vi "Butterfly_PullDown RCV w_AWG.vi"(0 "Semiconductor Module Context":T2, 1 "RFPins":string[](array[string]), 2 "script name":string, 3 "R Thresholds":dbl[](array[numeric]), 4 "Capacitance":bool=TRUE, 5 "error in (no error)":errorcluster, 6 "VNAs Measurement Parameters":T1, 7 "Start_v":dbl=10.0 format="%#_13g", 8 "C_TH_Delta":dbl=2.0, 9 "Stop_v":dbl=41.0 format="%#_13g", 10 "Down_Butterfly_V_Sweep":dbl[](array[numeric]), 11 "Step_v":dbl=1.0, 12 "DOWNPublishNames":string[](array[string])) -> (14 "Semiconductor Module Context Out":T2, 19 "error out":errorcluster)   [LabVIEW 2013]
uses:
  <vilib>/NI_TestStand_SemiconductorModule/NI_TestStand_Semiconductor_Module.lvlibp/PinMap/General/SemiconductorModuleContext.ctl
  VNA/VNAs Measurement Parameters.ctl
  <instrlib>/niHSDIO/niHSDIO.llb/niHSDIO_ctl Trigger Script - trigID Values (Ring).ctl
  <instrlib>/niDCPower/nidcpower.llb/niDCPower Wait For Event - Event.ctl
  <vilib>/NI_TestStand_SemiconductorModule/NI_TestStand_Semiconductor_Module.lvlibp/PinMap/DC Power/PinsToNIDCPowerSessions.vi
  <vilib>/NI_TestStand_SemiconductorModule/NI_TestStand_Semiconductor_Module.lvlibp/PinMap/General/Publish/PublishDataDoubleFunctionalTest.vi
  <vilib>/NI_TestStand_SemiconductorModule/NI_TestStand_Semiconductor_Module.lvlibp/PinMap/General/Publish/PublishDataDouble2D.vi
  <vilib>/NI_TestStand_SemiconductorModule/NI_TestStand_Semiconductor_Module.lvlibp
  VNA/Pin Map API/VNA Custom Instrument.lvlib
panel:
  in  "current level":dbl=0.01 format="%_6p"
  out "VPIs 2":dbl[](array[numeric])
  out "VRLs 2":dbl[](array[numeric])
  out "S0 steps":dbl[](array[numeric]) format="%#_3g"
  out "S1 steps":dbl[](array[numeric]) format="%#_3g"
  out "S2 steps":dbl[](array[numeric]) format="%#_3g"
  out "S3 steps":dbl[](array[numeric]) format="%#_3g"
  out "appended array":dbl[][](array[numeric]) format="%#_3g"
  out "VPIs":dbl[][](array[numeric]) format="%#_3g"
  out "VRLs":dbl[][](array[numeric]) format="%#_3g"
  out "C_Free":dbl[](array[numeric])
  out "Full R Array":dbl[][][](array[numeric])
  out "step":i32
  out "sites and pins loop iter":i32
  out "BF values":dbl[](array[numeric])
  out "BF Names":string[](array[string])
  out "R Array":dbl[](array[numeric])
  out "BFSamples":i32
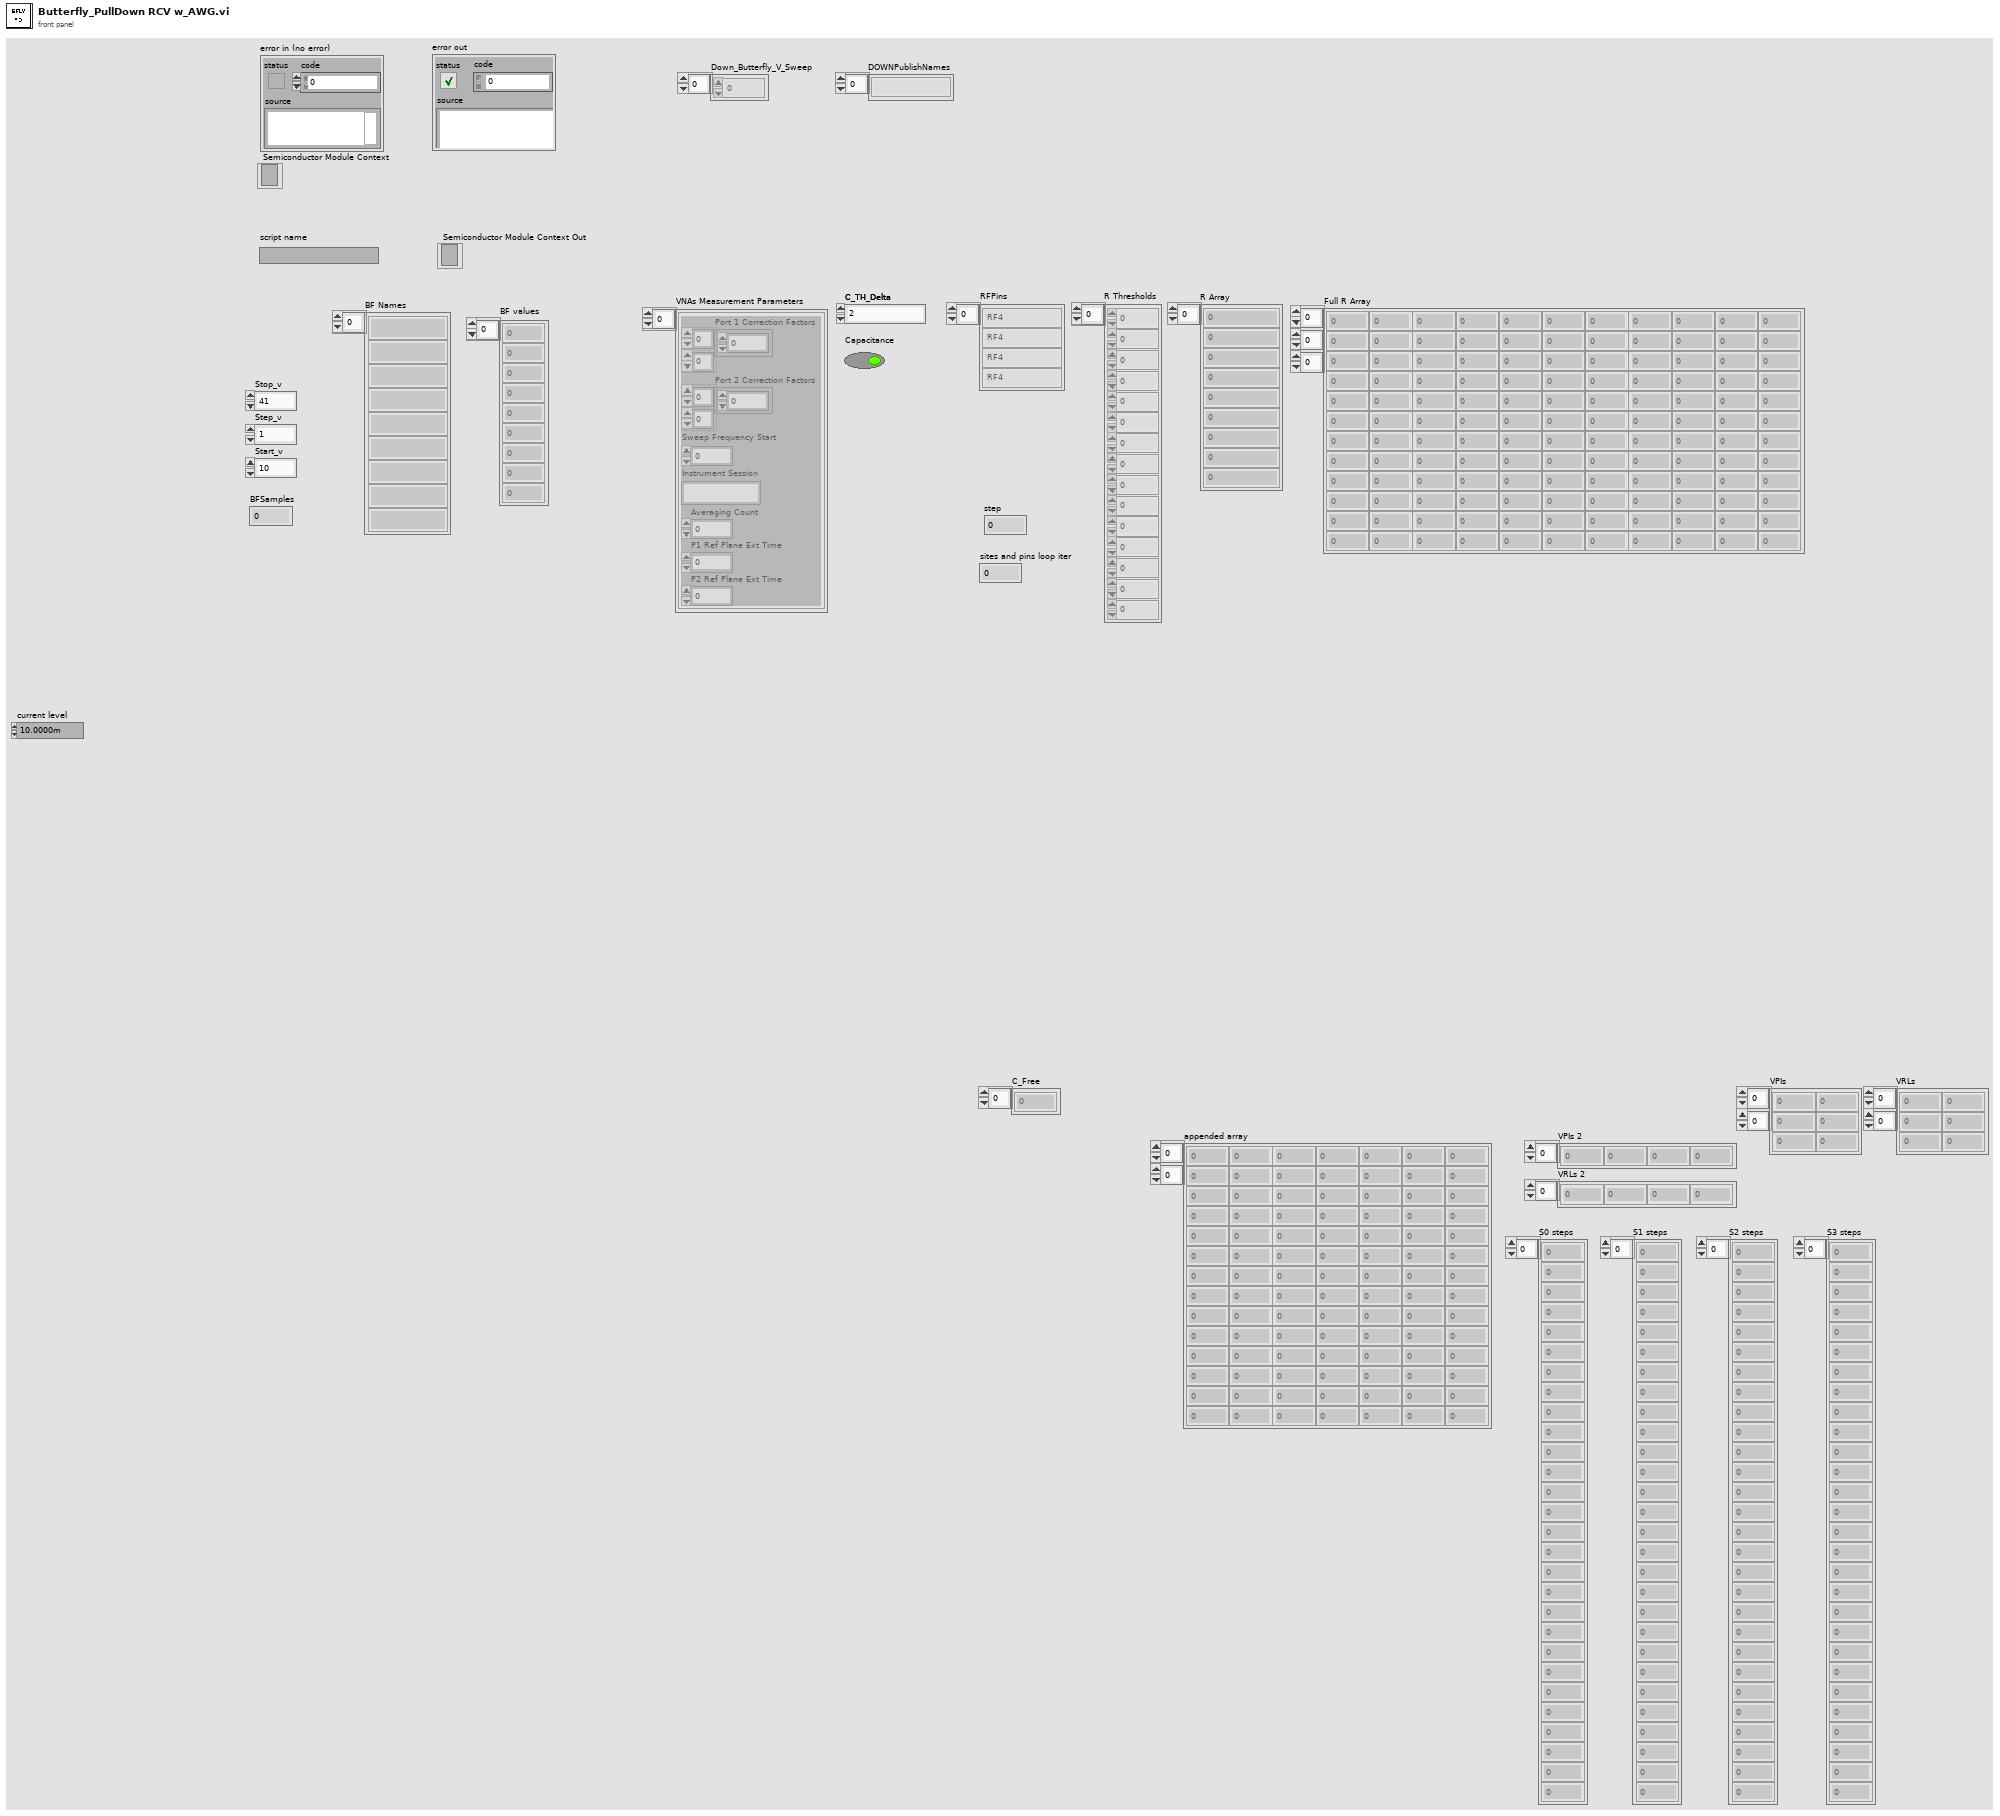
[diagram p1: front panel]
types:
  T1 = typedef "VNAs Measurement Parameters.ctl" = cluster{"Port 1 Correction Factors":cdb[][], "Port 2 Correction Factors":cdb[][], "Sweep Frequency Start":dbl, "Instrument Session":string, "Averaging Count":i32, "P1 Ref Plane Ext Time":dbl, "P2 Ref Plane Ext Time":dbl}[]
  T2 = typedef "NI_TestStand_Semiconductor_Module.lvlibp/SemiconductorModuleContext.ctl" = refnum<k7>
  T3 = typedef "niDCPower Wait For Event - Event.ctl" = i32
  T4 = typedef "niHSDIO_ctl Trigger Script - trigID Values (Ring).ctl" = string
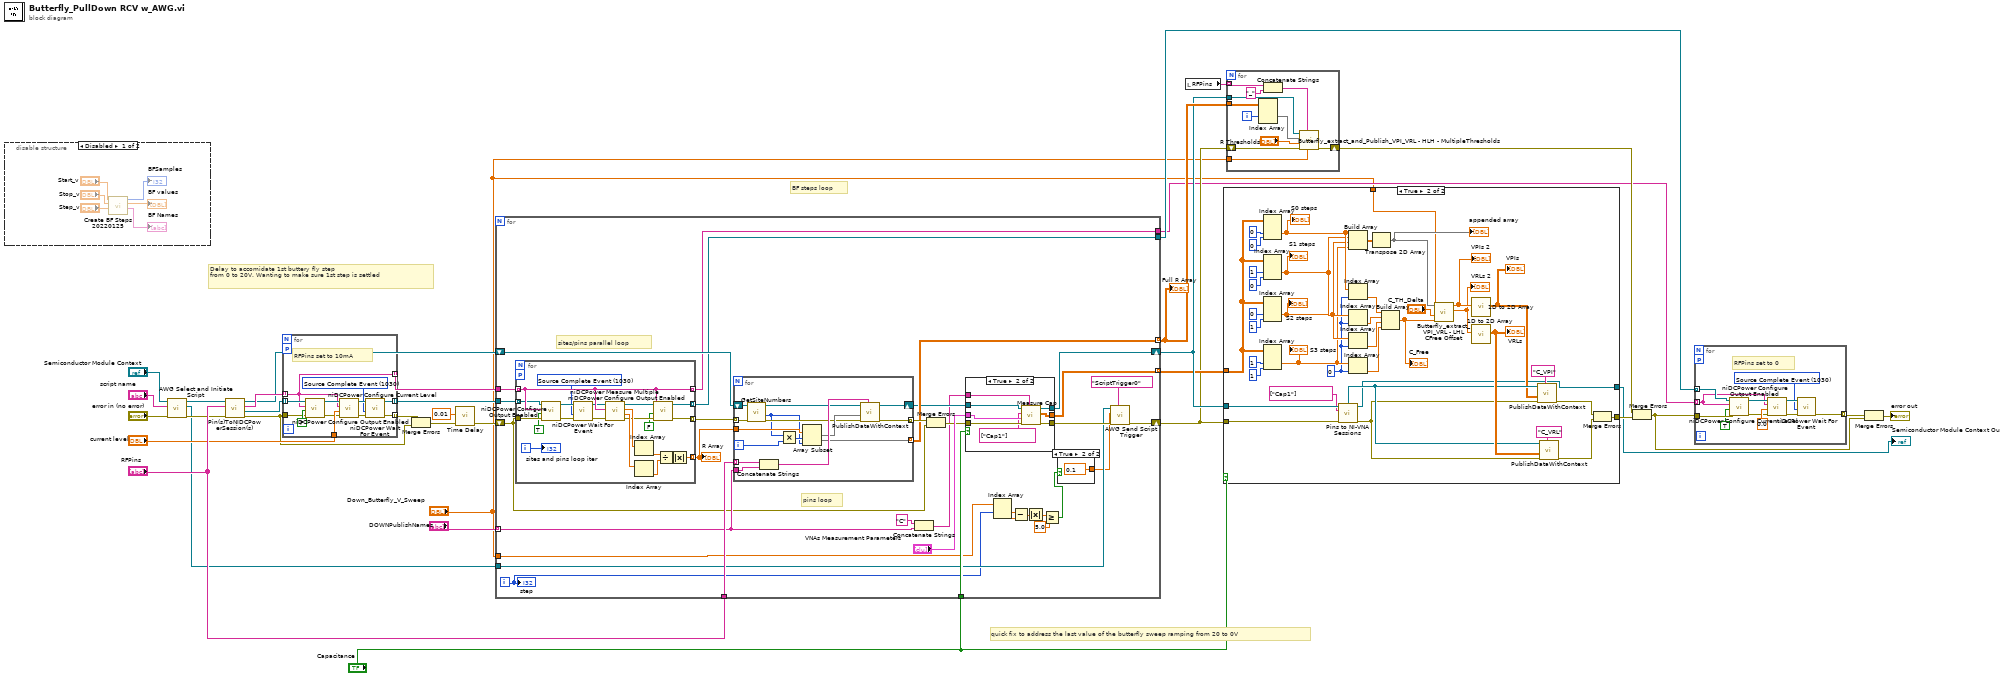
[diagram p0: block diagram]
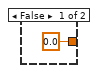
[diagram p4: hidden frame]
diagram:
  # "quick fix to address the last value of the butterfly sweep ramping from 20 to 0V"
  # "Delay to accomidate 1st buttery fly step\nfrom 0 to 20V. Wanting to make sure 1st step is settled"
  # "BF steps loop"
  n1 = disable-structure shown="Disabled" {
    frame Disabled {
      n2 = call "Create BF Steps 20220125.vi"("Step_v"="Step_v", "Stop_v"="Stop_v", "Start_v"="Start_v") -> ("BF Names"=→"BF Names":string[], "BF values"=→"BF values":dbl[], "BFSamples"=→"BFSamples":i32)  [unwired: 6 in]
    }
    frame Enabled {
    }
  }
  n3 = call "AWG Select and Initiate Script.vi"("error in (no error)"="error in (no error)", "script name"="script name", "Semiconductor Module Context"="Semiconductor Module Context") -> ("error out"=w10:errorcluster, "Sessions Out"=w6:refnum<k15>[], "Semiconductor Module Context Out"=w12:T2)  [unwired: 6 in]
  n4 = call-poly <vilib>:"Pin(s)ToNIDCPowerSession(s).vi"("error in (no error)"=w10, "Pins"="RFPins", "Semiconductor Module Context"=w12) -> ("error out"=w14:errorcluster, "Instrument Sessions"=w24:refnum<k15>[], "Channel Lists"=w23:string[], "Semiconductor Module Context Out"=w11:T2)  [unwired: 4 in, 1 out]
  n5 = for {
    tunnel: w24 -> [w47] mode=indexing
    tunnel: w23 -> [w43] mode=indexing
    tunnel: "current level" -> [w49]
    tunnel: [w42] -> w20 mode=indexing
    tunnel: [w43] -> w21 mode=indexing
    workers-P: _ -> [_]
    tunnel: w14 -> [w44]
    tunnel: [w41] -> w15 mode=indexing
    w50 = T3 1030 items=["Source Complete Event"=1030, "Measure Complete Event"=1031, "Sequence Iteration Complete Event"=1032, "Sequence Engine Done Event"=1033, "Pulse Complete Event"=1051, "Ready For Pulse Trigger Event"=1052] ("event")
    # "RFPins set to 10mA"
    n6 = call <instrlib>:"niDCPower Configure Output Enabled.vi"("error in (no error)"=w44, "output enabled"=FALSE, "channel name"=w43, "instrument handle"=w47) -> ("error out"=w45:errorcluster, "instrument handle out"=w46:refnum<k15>)  [unwired: 6 in]
    n7 = call <instrlib>:"niDCPower Configure Current Level.vi"("error in (no error)"=w45, "current level"=w49, "channel name"=w43, "instrument handle"=w46) -> ("error out"=w52:errorcluster, "instrument handle out"=w51:refnum<k15>)  [unwired: 6 in]
    n8 = call <instrlib>:"niDCPower Wait For Event.vi"("error in (no error)"=w52, "event"=w50, "instrument handle"=w51) -> ("error out"=w41:errorcluster, "instrument handle out"=w42:refnum<k15>)  [unwired: 7 in]
  }
  n9 = Merge Errors(w15, w14) -> (w5:errorcluster)
  n10 = call "Time Delay"("error in (no error)"=w5, "Delay Time (s)"=0.01) -> ("error out"=w4:errorcluster)  [unwired: 9 in]
  n11 = for {
    shift-right: [w61] -> w30
    shift-left: w4 -> [w66]
    shift-right: [w73] -> w32
    shift-left: w11 -> [w71]
    tunnel: "RFPins" -> [w84]
    tunnel: "DOWNPublishNames" -> [w76] mode=indexing
    tunnel: [w82] -> w33 mode=indexing
    tunnel: "Capacitance" -> [w74]
    tunnel: [w72] -> w31 mode=indexing
    tunnel: w21 -> [w70]
    tunnel: w20 -> [w69]
    tunnel: [w68] -> w19
    tunnel: [w67] -> w18
    tunnel: w6 -> [w63]
    tunnel: "Down_Butterfly_V_Sweep" -> [w60]
    i -> [w59]
    # "pins loop"
    # "sites/pins parallel loop"
    n12 = for {
      tunnel: w66 -> [w125]
      tunnel: [w127] -> w83 mode=indexing
      tunnel: [w123] -> w81 mode=indexing
      workers-P: _ -> [_]
      tunnel: w70 -> [w120] mode=indexing
      tunnel: w69 -> [w119] mode=indexing
      tunnel: [w121] -> w68 mode=indexing
      tunnel: [w120] -> w67 mode=indexing
      i -> [w126]
      w112 = T3 1030 items=["Source Complete Event"=1030, "Measure Complete Event"=1031, "Sequence Iteration Complete Event"=1032, "Sequence Engine Done Event"=1033, "Pulse Complete Event"=1051, "Ready For Pulse Trigger Event"=1052] ("event")
      n13 = call <instrlib>:"niDCPower Configure Output Enabled.vi"("error in (no error)"=w125, "output enabled"=TRUE, "channel name"=w120, "instrument handle"=w119) -> ("error out"=w116:errorcluster, "instrument handle out"=w113:refnum<k15>)  [unwired: 6 in]
      n14 = call <instrlib>:"niDCPower Wait For Event.vi"("error in (no error)"=w116, "event"=w112, "instrument handle"=w113) -> ("error out"=w115:errorcluster, "instrument handle out"=w114:refnum<k15>)  [unwired: 7 in]
      n15 = call <instrlib>:"niDCPower Measure Multiple.vi"("error in (no error)"=w115, "channel name"=w120, "instrument handle"=w114) -> ("error out"=w124:errorcluster, "current measurements"=w128:dbl[], "voltage measurements"=w129:dbl[], "instrument handle out"=w122:refnum<k15>)  [unwired: 5 in]
      n16 = Index Array(array=w129) -> (element=w131:dbl)  [unwired: 1 in]
      n17 = Index Array(array=w128) -> (element=w130:dbl)  [unwired: 1 in]
      n18 = call <instrlib>:"niDCPower Configure Output Enabled.vi"("error in (no error)"=w124, "output enabled"=FALSE, "channel name"=w120, "instrument handle"=w122) -> ("error out"=w123:errorcluster, "instrument handle out"=w121:refnum<k15>)  [unwired: 6 in]
      n19 = Divide(x=w131, y=w130) -> (x/y=w132:dbl)
      n20 = Absolute Value(x=w132) -> (abs(x)=w127:dbl)
      "sites and pins loop iter" <- w126
    }
    "R Array" <- w83
    n21 = for {
      tunnel: [w106] -> w85 mode=indexing
      tunnel: w84 -> [w110] mode=indexing
      tunnel: w83 -> [w107]
      tunnel: w76 -> [w109]
      shift-right: [w104] -> w80
      shift-left: w71 -> [w101]
      tunnel: [w103] -> w82 mode=indexing
      tunnel: w81 -> [w98] mode=indexing
      i -> [w111]
      n22 = call <vilib>:"GetSiteNumbers.vi"("error in (no error)"=w98, "Semiconductor Module Context"=w101) -> ("error out"=w102:errorcluster, "Number Of Sites"=w99:i32, "Semiconductor Module Context Out"=w100:T2)  [unwired: 6 in, 1 out]
      n23 = Concatenate Strings(w110, w109) -> (w105:string)
      n24 = Multiply(x=w99, y=w111) -> (x*y=w108:i32)
      n25 = Array Subset(array=w107, index=w108, length=w99) -> (w103:dbl[])
      n26 = call-poly <vilib>:"PublishDataWithContext.vi"("Published Data Id"=w105, "error in (no error)"=w102, "Data In"=w103, "Semiconductor Module Context"=w100) -> ("error out"=w106:errorcluster, "Semiconductor Module Context Out"=w104:T2)  [unwired: 6 in]
    }
    n27 = Concatenate Strings("C" ("string"), w76) -> (w75:string)
    n28 = Merge Errors(w85, w66) -> (w78:errorcluster)
    n29 = case shown="True" w74 {
      tunnel: w80 -> [w89 w97]
      tunnel: [w89 w96] -> w73
      tunnel: [w88 w94] -> w65
      tunnel: w75 -> [_ w90]
      tunnel: "VNAs Measurement Parameters" -> [_ w92]
      tunnel: [_ w93] -> w72
      tunnel: w78 -> [w88 w95]
      frame False {
      }
      frame True {
        n30 = call "Measure Cap.vi"("Measurement Id"=w90, "error in (no error)"=w95, "VNAs Measurement Parameters"=w92, "Pins"=string[] ["Cap1"] ("Capacitance Pins"), "Semiconductor Module Context"=w97) -> ("error out"=w94:errorcluster, "Multisite Cap Data"=w93:dbl[][], "Semiconductor Module Context Out"=w96:T2)  [unwired: 4 in]
      }
    }
    n31 = Index Array(array=w60, index #1=w59) -> (element #1=w58:dbl, element #2=w57:dbl)  [unwired: 1 in]
    n32 = Subtract(x=w58, y=w57) -> (x-y=w56:dbl)
    n33 = Absolute Value(x=w56) -> (abs(x)=w55:dbl)
    n34 = Greater Or Equal?(x=w55, y=5.0) -> (x >= y?=w53:bool)
    n35 = case shown="True" w53 {
      tunnel: [0.0 ("Delay Time (s)") 0.1 ("Delay Time (s)")] -> w62
      frame False {
      }
      frame True {
      }
    }
    n36 = call "AWG Send Script Trigger.vi"("trigger id (script trigger 0)"=T4 "ScriptTrigger0", "error in (no error)"=w65, "Delay Time (s)"=w62, "AWG Sessions In"=w63) -> ("error out"=w61:errorcluster)  [unwired: 6 in, 1 out]
    "step" <- w59
  }
  "Full R Array" <- w33
  n37 = local read "RFPins"() -> (w34:string[])
  n38 = case shown="True" "Capacitance" {
    tunnel: [w133 w153] -> w26
    tunnel: [w134 w171] -> w27
    tunnel: w32 -> [w133 w170]
    tunnel: w30 -> [w134 w166]
    tunnel: "Down_Butterfly_V_Sweep" -> [_ w138]
    tunnel: w31 -> [_ w157]
    frame False {
    }
    frame True {
      w146 = 0 ("index")
      n39 = Index Array(array=w157, index (dim 1)=0 ("disabled index (row)"), index (dim 2)=0 ("disabled index (col)")) -> (element=w150:dbl[])  [unwired: 1 in]
      "S0 steps" <- w150
      n40 = Index Array(array=w157, index (dim 1)=1 ("index (row)"), index (dim 2)=0 ("index (col)")) -> (element=w149:dbl[])  [unwired: 1 in]
      "S1 steps" <- w149
      n41 = Index Array(array=w157, index (dim 1)=0 ("index (row)"), index (dim 2)=1 ("index (col)")) -> (element=w148:dbl[])  [unwired: 1 in]
      "S2 steps" <- w148
      n42 = Index Array(array=w157, index (dim 1)=1 ("index (row)"), index (dim 2)=1 ("index (col)")) -> (element=w147:dbl[])  [unwired: 1 in]
      "S3 steps" <- w147
      n43 = call "Pins to NI-VNA Sessions.vi"("Semiconductor Module Context"=w170, "Pins"=string[] ["Cap1"] ("Capacitance Pins"), "error in (no error)"=w166) -> ("Pin Query Context"=w156:refnum<class "MultiplePinMultipleSessionQueryContext.lvclass">, "Semiconductor Module Context Out"=w153:T2, "error out"=w151:errorcluster)  [unwired: 8 in, 2 out]
      n44 = Build Array(w150, w149, w148, w147) -> (w141:dbl[][])
      n45 = Index Array(array=w150, index=w146) -> (element=w145:dbl)
      n46 = Index Array(array=w149, index=w146) -> (element=w144:dbl)
      n47 = Index Array(array=w148, index=w146) -> (element=w143:dbl)
      n48 = Index Array(array=w147, index=w146) -> (element=w142:dbl)
      n49 = Transpose 2D Array(2D array=w141) -> (transposed array=w139:dbl[][])
      "appended array" <- w139
      n50 = Build Array(w145, w144, w143, w142) -> (w140:dbl[])
      "C_Free" <- w140
      n51 = call "Butterfly_extract_VPI_VRL - LHL CFree Offset.vi"("C_Free"=w140, "Delta"="C_TH_Delta", "Voltage Array"=w138, "Result Array In"=w139) -> ("VRLs"=w135:dbl[], "VPIs"=w136:dbl[])  [unwired: 6 in]
      "VPIs 2" <- w136
      "VRLs 2" <- w135
      n52 = call "1D to 2D Array.vi"("1D Array"=w136) -> ("2D Array"=w155:dbl[][])  [unwired: 10 in]
      "VPIs" <- w155
      n53 = call "1D to 2D Array.vi"("1D Array"=w135) -> ("2D Array"=w169:dbl[][])  [unwired: 10 in]
      "VRLs" <- w169
      n54 = call-poly <vilib>:"PublishDataWithContext.vi"("Published Data Id"="C_VPI", "error in (no error)"=w151, "Data In"=w155, "Pin Query Context"=w156) -> ("error out"=w152:errorcluster)  [unwired: 6 in, 1 out]
      n55 = call-poly <vilib>:"PublishDataWithContext.vi"("Published Data Id"="C_VRL", "error in (no error)"=w151, "Data In"=w169, "Pin Query Context"=w156) -> ("error out"=w172:errorcluster)  [unwired: 6 in, 1 out]
      n56 = Merge Errors(w152, w172) -> (w171:errorcluster)
    }
  }
  "Semiconductor Module Context Out" <- w26
  n57 = for {
    tunnel: w34 -> [w177] mode=indexing
    tunnel: w33 -> [w182]
    shift-right: [w178] -> w28
    shift-left: w30 -> [w179]
    tunnel: w32 -> [w174]
    tunnel: "Down_Butterfly_V_Sweep" -> [w173]
    i -> [w183]
    n58 = Index Array(array=w182, index (dim 1)=w183) -> (element=w180:dbl[][])  [unwired: 2 in]
    n59 = Concatenate Strings(w177, "_" ("string")) -> (w175:string)
    n60 = call "Butterfly_extract_and_Publish_VPI_VRL - HLH - MultipleThresholds.vi"("Voltages Array"=w173, "ID Prefix"=w175, "error in (no error)"=w179, "Thresholds"="R Thresholds", "Result Array In"=w180, "Semiconductor Module Context"=w174) -> ("error out"=w178:errorcluster)  [unwired: 5 in]
  }
  n61 = Merge Errors(w28, w27) -> (w7:errorcluster)
  n62 = for {
    tunnel: w19 -> [w187] mode=indexing
    tunnel: w18 -> [w185] mode=indexing
    workers-P: _ -> [_]
    tunnel: w7 -> [w189]
    tunnel: [w191] -> w17 mode=indexing
    w190 = T3 1030 items=["Source Complete Event"=1030, "Measure Complete Event"=1031, "Sequence Iteration Complete Event"=1032, "Sequence Engine Done Event"=1033, "Pulse Complete Event"=1051, "Ready For Pulse Trigger Event"=1052] ("event")
    # "RFPins set to 0"
    n63 = call <instrlib>:"niDCPower Configure Output Enabled.vi"("error in (no error)"=w189, "output enabled"=TRUE, "channel name"=w185, "instrument handle"=w187) -> ("error out"=w188:errorcluster, "instrument handle out"=w186:refnum<k15>)  [unwired: 6 in]
    n64 = call <instrlib>:"niDCPower Configure Current Level.vi"("error in (no error)"=w188, "current level"=0.0, "channel name"=w185, "instrument handle"=w186) -> ("error out"=w194:errorcluster, "instrument handle out"=w193:refnum<k15>)  [unwired: 6 in]
    n65 = call <instrlib>:"niDCPower Wait For Event.vi"("error in (no error)"=w194, "event"=w190, "instrument handle"=w193) -> ("error out"=w191:errorcluster)  [unwired: 7 in, 1 out]
  }
  n66 = Merge Errors(w17, w7) -> (→"error out":errorcluster)
